vi "RxTx.vi"(8 "error in (no error)":errorcluster) -> (0 "error out":errorcluster)   [LabVIEW 2018]
uses:
  RxTx/RxTx.lvclass
  <vilib>/addons/_JKI Toolkits/Caraya/classes/Assert/Assert Equal Value_Variant.vi
  <vilib>/addons/_JKI Toolkits/Caraya/classes/Test/Test.lvclass
  <vilib>/addons/_JKI Toolkits/Caraya/classes/Assert/Assert.lvclass
panel:
  in  "RxTx in":refnum<class "RxTx.lvclass">
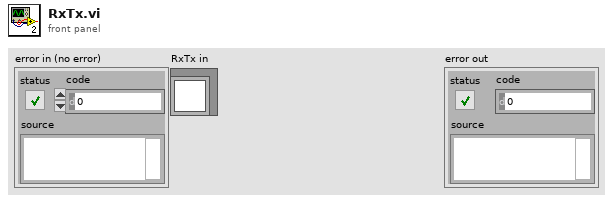
[diagram p1: front panel]
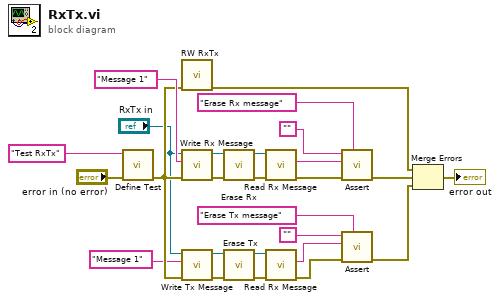
[diagram p0: block diagram]
diagram:
  n1 = call <vilib>:"Define Test.vi"("error in (no error)"="error in (no error)", "Label (VI Title)"="Test RxTx") -> ("error out"=w4:errorcluster)  [unwired: 8 in, 1 out]
  n2 = call "RW RxTx.vi"("error in (no error)"=w4) -> ("error out"=w24:errorcluster)  [unwired: 10 in]
  n3 = call "Write Rx Message.vi"("error in (no error)"=w4, "Rx Message"="Message 1", "RxTx in"="RxTx in") -> ("error out"=w22:errorcluster, "RxTx out"=w21:refnum<class "RxTx.lvclass">)  [unwired: 7 in]
  n4 = call "Write Tx Message.vi"("error in (no error)"=w4, "Tx Message"="Message 1" ("Rx Message"), "RxTx in"="RxTx in") -> ("error out"=w8:errorcluster, "RxTx out"=w7:refnum<class "RxTx.lvclass">)  [unwired: 7 in]
  n5 = call "Erase Rx.vi"("error in (no error)"=w22, "RxTx in"=w21) -> ("error out"=w20:errorcluster, "RxTx out"=w15:refnum<class "RxTx.lvclass">)  [unwired: 8 in]
  n6 = call "Erase Tx.vi"("error in (no error)"=w8, "RxTx in"=w7) -> ("error out"=w5:errorcluster, "RxTx out"=w6:refnum<class "RxTx.lvclass">)  [unwired: 8 in]
  n7 = call "Read Rx Message.vi"("error in (no error)"=w20, "RxTx in"=w15) -> ("error out"=w19:errorcluster, "Rx Message"=w18:string)  [unwired: 7 in, 1 out]
  n8 = call "Read Rx Message.vi"("error in (no error)"=w5, "RxTx in"=w6) -> ("error out"=w9:errorcluster, "Rx Message"=w10:string)  [unwired: 7 in, 1 out]
  n9 = call-poly <vilib>:"Assert.vi"("Label"="Erase Rx message" ("Label (VI Title)"), "error in (no error)"=w19, "Y"=w18, "X"="") -> ("error out"=w14:errorcluster)  [unwired: 6 in, 1 out]
  n10 = call-poly <vilib>:"Assert.vi"("Label"="Erase Tx message" ("Label (VI Title)"), "error in (no error)"=w9, "Y"=w10, "X"="") -> ("error out"=w2:errorcluster)  [unwired: 6 in, 1 out]
  n11 = Merge Errors(w24, w14, w2) -> (→"error out":errorcluster)
